vi "Write Query TDM.vi"(6 "Max Results (-1 is ALL)":i32=-1, 8 "error in (no error)":errorcluster, 9 "DataFinder parameters":T2[](array[typedef]), 10 "Return Type (ChannelGroup)":T1=enum."eSearchChannelGroup", 11 "Query Path":path) -> (0 "error out":errorcluster, 3 "Query Path Out":path)   [LabVIEW 2011]
uses:
  <vilib>/Platform/storage/lvStorage.llb/xStorage/Write Data/Write Data.xnode
  <vilib>/Platform/storage/lvStorage.llb/_createOrGetByNameExplicitChildObject.vi
  <vilib>/Platform/storage/Storage.llb/__savePropString.vi
  <vilib>/Platform/storage/lvStorage.llb/xStorage/xStorageSupp/ErrorOut.vi
  <vilib>/Platform/storage/lvStorage.llb/_saveStringChannel.vi
  <vilib>/Platform/storage/Storage.llb/usiSequenceRepresentation.ctl
  eSearch Types.ctl
  DataFinder Comparisons.ctl
  Datafinder Query.ctl
panel:
  out "Condition Array":string[][](array[string])
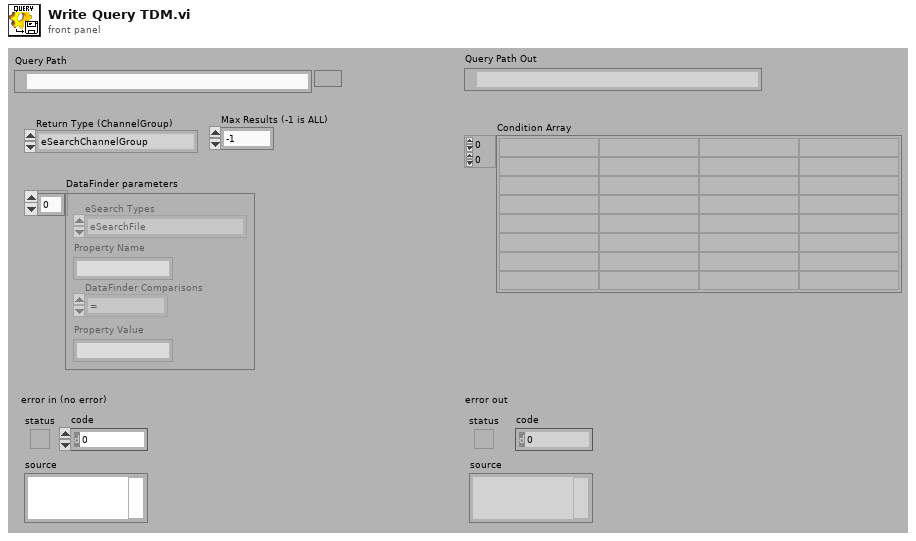
[diagram p1: front panel]
types:
  T1 = typedef "eSearch Types.ctl" = enum16{"eSearchFile", "eSearchChannelGroup", "eSearchChannel"}
  T2 = typedef "Datafinder Query.ctl" = cluster{"eSearch Types":T1, "Property Name":string, "DataFinder Comparisons":T3, "Property Value":string}
  T3 = typedef "DataFinder Comparisons.ctl" = enum16{"=", "<>", "<", "<=", ">", ">="}
  T4 = enum16{"UPDATE", "READ", "QUERY", "CREATE CHILD", "CREATE", "CONNECT", "DISCONNECT"}
  T5 = enum16{"Append values", "Replace values at index", "Replace all values"}
  T6 = typedef "usiSequenceRepresentation.ctl" = enum16{"explicit", "implicit"}
  T7 = enum16{"open", "open or create", "create or replace", "create", "open (read only)"}
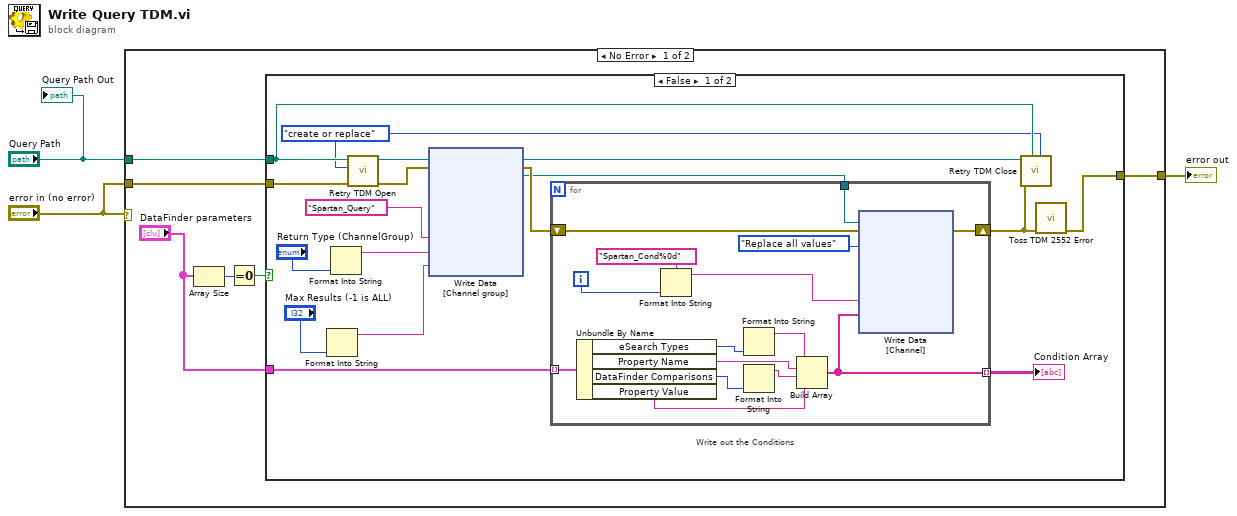
[diagram p0: block diagram]
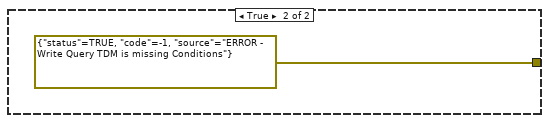
[diagram p2: hidden frame]
diagram:
  n1 = case shown="No Error" "error in (no error)" {
    tunnel: "Query Path" -> [w9 _]
    tunnel: "error in (no error)" -> [w8 w84]
    tunnel: [w7 w84] -> w2
    frame No Error {
      n2 = Array Size(array="DataFinder parameters") -> (size(s)=w5:i32)
      n3 = Equal To 0?(x=w5) -> (x = 0?=w4:bool)
      n4 = case shown="False" w4 {
        tunnel: w9 -> [w14 _]
        tunnel: w8 -> [w20 _]
        tunnel: "DataFinder parameters" -> [w24 _]
        tunnel: [w15 errorcluster {"status"=TRUE, "code"=-1, "source"="ERROR - Write Query TDM is missing Conditions"} ("error out")] -> w7
        frame False {
          w13 = T7."create or replace" ("function (open:0)")
          # "Write out the Conditions"
          n5 = Format Into String("Max Results (-1 is ALL)") -> (resulting string=w16:string)  [unwired: 3 in, 1 out]
          n6 = Format Into String("Return Type (ChannelGroup)") -> (resulting string=w23:string)  [unwired: 3 in, 1 out]
          n7 = call "Retry TDM Open.vi"("error in"=w20, "function (open:0)"=w13, "Path"=w14) -> ("error out"=w19:errorcluster, "storage refnum (file)"=w18:refnum<k20>)  [unwired: 7 in]
          n8 = xnode "Write Data\n[Channel group]"("Name"="Spartan_Query", "Description"=w23, "Free text 1"=w16, "storage refnum (file)"=w18, "error in"=w19) -> ("storage refnum (file) out"=w10:refnum<k20>, "error out"=w25:errorcluster, "storage refnum (channel group)"=w12:refnum<k20>)
          n9 = for {
            tunnel: w12 -> [w60]
            shift-right: [w59] -> w11
            shift-left: w25 -> [w62]
            tunnel: w24 -> [w58] mode=indexing
            tunnel: [w48] -> w21 mode=indexing
            i -> [w50]
            n10 = Unbundle By Name(w58) -> ("eSearch Types"=w57:T1, "Property Name"=w55:string, "DataFinder Comparisons"=w54:T3, "Property Value"=w52:string)
            n11 = Format Into String(format string="Spartan_Cond%0d", w50) -> (resulting string=w49:string)  [unwired: 2 in, 1 out]
            n12 = Format Into String(w57) -> (resulting string=w56:string)  [unwired: 3 in, 1 out]
            n13 = Format Into String(w54) -> (resulting string=w53:string)  [unwired: 3 in, 1 out]
            n14 = Build Array(w56, w55, w53, w52) -> (w48:string[])
            n15 = xnode "Write Data\n[Channel]"("Name"=w49, "Signal"=w48, "storage refnum (channel group)"=w60, "error in"=w62, "append / replace (append data values)"=T5."Replace all values") -> ("error out"=w59:errorcluster)  [unwired: 1 in, 2 out]
          }
          "Condition Array" <- w21
          n16 = call "Retry TDM Close.vi"("function (open:0)"=w13, "TDM Path"=w14, "error in"=w11, "storage refnum (file)"=w10) -> ()  [unwired: 7 in, 1 out]
          n17 = call "Toss TDM 2552 Error.vi"("error in (no error)"=w11) -> ("error out"=w15:errorcluster)  [unwired: 10 in]
        }
        frame True {
        }
      }
    }
    frame Error {
    }
  }
  "error out" <- w2
  "Query Path Out" <- "Query Path"
